vi "create Behaviour.vi"(8 "error in (no error)":errorcluster caption="Fehler (Eingang, kein Fehler)", 11 "Spannungseinbruch Eingang":refnum<class "Spannungseinbruch.lvclass"> caption="DNL_LabVIEW Object in") -> (0 "error out":errorcluster caption="Fehler (Ausgang)", 1 "regex":string[](array[string]), 2 "response":bool[](array[boolean]), 3 "Spannungseinbruch Ausgang":refnum<class "Spannungseinbruch.lvclass"> caption="DNL_LabVIEW Object out")   [LabVIEW 2013, in "Spannungseinbruch.lvclass"]
uses:
  Spannungseinbruch.lvclass
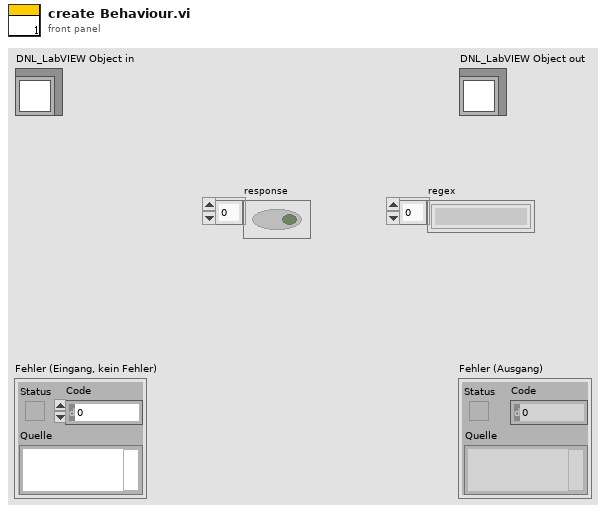
[diagram p1: front panel]
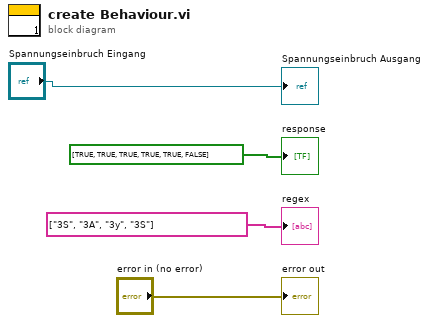
[diagram p0: block diagram]
diagram:
  "error out" <- "error in (no error)"
  "Spannungseinbruch Ausgang" <- "Spannungseinbruch Eingang"
  "regex" <- string[] ["3S", "3A", "3y", "3S"]
  "response" <- bool[] [TRUE, TRUE, TRUE, TRUE, TRUE, FALSE]
